vi "IBM4_Read(VN).vi"(8 "error in":errorcluster, 9 "Number":i32=10, 10 "Channel":i32=3 min=0 max=4, 11 "COM resource in":refnum<visa-resource-name>="ASRL5::INSTR") -> (0 "error out":errorcluster, 2 "array":dbl[](array[numeric]), 3 "COM resource out":refnum<visa-resource-name>="ASRL5::INSTR")   [LabVIEW 2021, in "IBM4.lvlib"]
doc: "This VI interfaces with the IBM4 to perform a read operation.\n\nThe input channel must be between 0 and 3, And the number of readings should be greater than zero. At some point the number of reading will be too high and will cause a timeout error. This should only happen for numbers larger than 10000. The output will be an array of floating point (Voltage) values.\n\nAlternate read operations exist covering binary or floating point, single reading, multiple readings, and an average of multiple readings (floating point only)."
uses:
  <instrlib>/IBM4/IBM4.lvlib
  <vilib>/Instr/_visa.llb/VISA Configure Serial Port (Instr).vi
panel:
  out "Array":u32[](array[numeric])
  out "read buffer":string="Output 3 = 1.85786 \r\n"
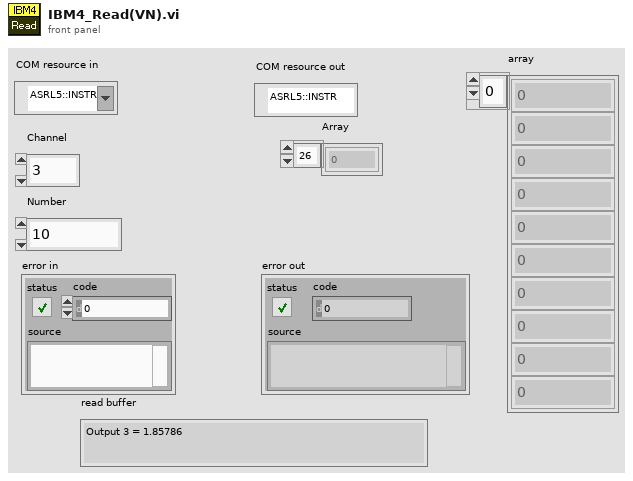
[diagram p1: front panel]
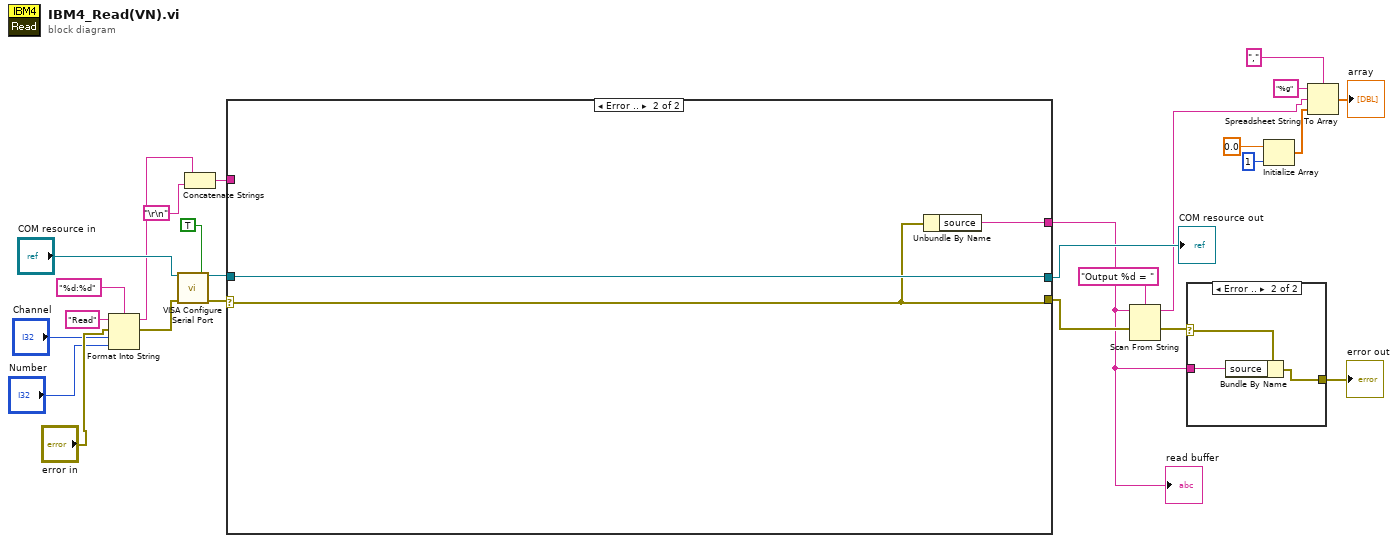
[diagram p0: block diagram]
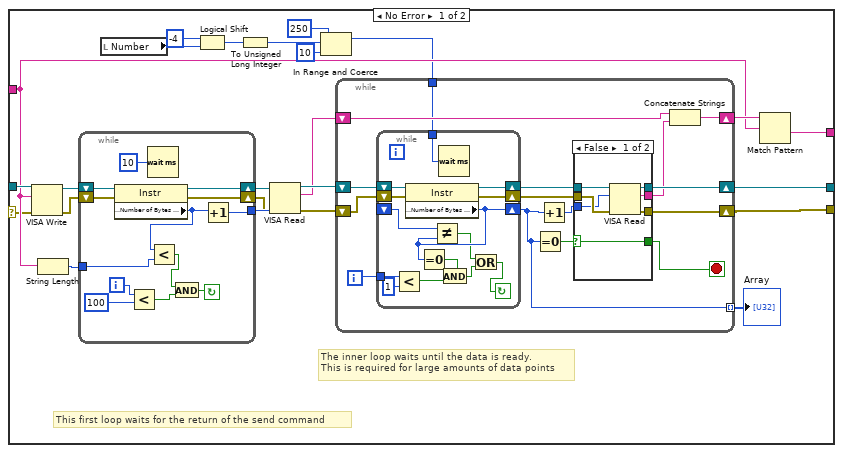
[diagram p3: hidden frame]
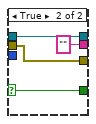
[diagram p4: hidden frame]
diagram:
  n1 = Format Into String(format string="%d:%d", initial string="Read", error in="error in", "Channel", "Number") -> (resulting string=w12:string, error out=w21:errorcluster)
  n2 = call-poly "VISA Configure Serial Port"("VISA resource name"="COM resource in", "Enable Termination\nChar (T)"=TRUE ("Enable Termination\nChar (T)"), "error in (no error)"=w21) -> ("VISA resource name out"=w18:refnum<visa-resource-name>, "error out"=w17:errorcluster)  [unwired: 11 in]
  n3 = Concatenate Strings(w12, "\r\n") -> (w11:string)
  n4 = case shown="Error .." w17 {
    selector: w17 -> [w37 w105]
    tunnel: w18 -> [w50 w106]
    tunnel: [w36 w105] -> w15
    tunnel: [w48 w104] -> w8
    tunnel: w11 -> [w47 _]
    tunnel: [w35 w106] -> w16
    frame No Error {
      # "The inner loop waits until the data is ready.\nThis is required for large amounts of data points"
      # "This first loop waits for the return of the send command"
      n5 = VISA Write(VISA resource name=w50, write buffer=w47, error in (no error)=w37) -> (VISA resource name out=w46:refnum<visa-resource-name>, error out=w45:errorcluster)  [unwired: 1 out]
      n6 = String Length(string=w47) -> (length=w38:i32)
      n7 = while {
        tunnel: [w52] -> w43
        shift-right: [w62] -> w44
        shift-left: w46 -> [w63]
        shift-right: [w60] -> w42
        shift-left: w45 -> [w61]
        tunnel: w38 -> [w58]
        i -> [w53]
        stop <- w56 continue-if-true
        n8 = property class="Instr"(reference=w63, error in=w61) -> (reference out=w62:refnum<visa-resource-name>, error out=w60:errorcluster, "Serial Settings:Number of Bytes at Serial Port"=w51:u32)
        n9 = Less?(x=w53, y=100) -> (x < y?=w55:bool)
        n10 = Wait (ms)(milliseconds to wait=u32 10) -> ()  [unwired: 1 out]
        n11 = Less?(x=w51, y=w58) -> (x < y?=w54:bool)
        n12 = And(x=w54, y=w55) -> (x .and. y?=w56:bool)
        n13 = Increment(x=w51) -> (x+1=w52:u32)
      }
      n14 = local read "Number"() -> (w30:i32)
      n15 = Logical Shift(y=i16 -4, x=w30) -> (x << y=w31:i32)
      n16 = To Unsigned Long Integer(number=w31) -> (unsigned 32bit integer=w28:u32)
      n17 = VISA Read(VISA resource name=w44, byte count=w43, error in (no error)=w42) -> (VISA resource name out=w41:refnum<visa-resource-name>, read buffer=w39:string, error out=w40:errorcluster)  [unwired: 1 out]
      n18 = In Range and Coerce(upper limit=u32 250, x=w28, lower limit=u32 10) -> (coerced(x)=w27:u32)  [unwired: 1 out]
      n19 = while {
        shift-right: [w78] -> w35
        shift-left: w41 -> [w76]
        shift-right: [w77] -> w36
        shift-left: w40 -> [w74]
        shift-right: [w72] -> w49
        shift-left: w39 -> [w70]
        tunnel: [w65] -> w34 mode=indexing
        tunnel: w27 -> [w64]
        i -> [w69]
        stop <- w66 stop-if-true
        n20 = while {
          shift-right: [w102] -> w75
          shift-left: w76 -> [w103]
          shift-right: [w100] -> w73
          shift-left: w74 -> [w101]
          tunnel: w69 -> [w99]
          shift-right: [w95] -> w65
          shift-left: _ -> [w94]
          tunnel: w64 -> [w90]
          stop <- w91 continue-if-true
          n21 = Less?(x=w99, y=1) -> (x < y?=w97:bool)
          n22 = property class="Instr"(reference=w103, error in=w101) -> (reference out=w102:refnum<visa-resource-name>, error out=w100:errorcluster, "Serial Settings:Number of Bytes at Serial Port"=w95:u32)
          n23 = Equal To 0?(x=w95) -> (x = 0?=w96:bool)
          n24 = Not Equal?(x=w94, y=w95) -> (x != y?=w92:bool)
          n25 = Wait (ms)(milliseconds to wait=w90) -> ()  [unwired: 1 out]
          n26 = And(x=w96, y=w97) -> (x .and. y?=w93:bool)
          n27 = Or(x=w92, y=w93) -> (x .or. y?=w91:bool)
        }
        n28 = Equal To 0?(x=w65) -> (x = 0?=w67:bool)
        n29 = Increment(x=w65) -> (x+1=w68:u32)
        n30 = case shown="False" w67 {
          selector: w67 -> [w79 w88]
          tunnel: [w85 w89] -> w78
          tunnel: [w84 w87] -> w77
          tunnel: w75 -> [w83 w89]
          tunnel: w73 -> [w82 w87]
          tunnel: [w81 "" ("read buffer")] -> w71
          tunnel: w68 -> [w80 _]
          tunnel: [w79 w88] -> w66
          frame False {
            n31 = VISA Read(VISA resource name=w83, byte count=w80, error in (no error)=w82) -> (VISA resource name out=w85:refnum<visa-resource-name>, read buffer=w81:string, error out=w84:errorcluster)  [unwired: 1 out]
          }
          frame True {
          }
        }
        n32 = Concatenate Strings(w70, w71) -> (w72:string)
      }
      "Array" <- w34
      n33 = Match Pattern(string=w49, regular expression=w47) -> (after substring=w48:string)  [unwired: 1 in, 3 out]
    }
    frame Error {
      n34 = Unbundle By Name(w105) -> ("source"=w104:string)
    }
  }
  "COM resource out" <- w16
  "read buffer" <- w8
  n35 = Scan From String(format string="Output %d = ", input string=w8, error in=w15) -> (remaining string=w2:string, error out=w10:errorcluster)  [unwired: 3 in, 1 out]
  n36 = case shown="Error .." w10 {
    selector: w10 -> [w107 w110]
    tunnel: [w107 w108] -> w9
    tunnel: w8 -> [_ w109]
    frame No Error {
    }
    frame Error {
      n37 = Bundle By Name(cluster=w110, "source"=w109) -> (w108:errorcluster)
    }
  }
  "error out" <- w9
  n38 = Initialize Array(0.0, 1 ("dimension size")) -> (w6:dbl[])
  n39 = Spreadsheet String To Array(delimiter (Tab)=",", format string="%g", spreadsheet string=w2, array type (2D Dbl)=w6) -> (array=→"array":dbl[])
